vi "open device.vi"(8 "error in (no error)":errorcluster, 11 "name":string) -> (0 "error out":errorcluster, 3 "function return":i32)   [LabVIEW 2012, in "libximc.lvlib"]
doc: "device_t XIMC_API open_device (const char* name);"
uses:
  libximc.lvlib
  libximc.dll
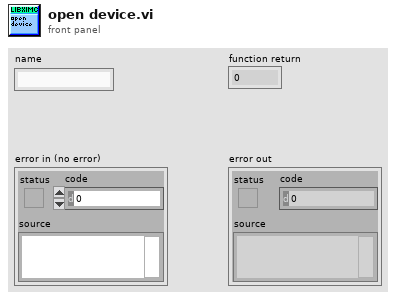
[diagram p1: front panel]
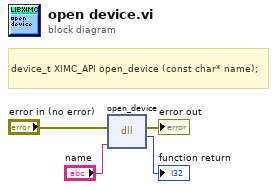
[diagram p0: block diagram]
diagram:
  # "device_t XIMC_API open_device (const char* name);"
  n1 = dll-call lib="C:/Users/user/Desktop/labview-2.9.11-gen/libximc.*" fn="open_device"(error in="error in (no error)", "name"="name") -> (error out=→"error out":errorcluster, →"function return":i32)  [unwired: 3 in, 1 out]
